vi "enqeue.vi"(9 "memory ref":refnum<k21>, 10 "data":u16, 11 "buffer state in":T1) -> (3 "buffer state out":T1)   [LabVIEW 2010, in "OnBoardBuffer.lvlib"]
uses:
  OnBoardBuffer.lvlib
  buffer_state_cluster.ctl
  <vilib>/rvi/DataTransferAndStorage/Container/XNode/niFpgaContainer.xnode
  <vilib>/rvi/DataTransferAndStorage/Container/Common/niFpgaContainerMetaDataKey.ctl
  <vilib>/rvi/DataTransferAndStorage/Container/Common/niFpgaContainerExecOnDevCompGetState.vi
  <vilib>/rvi/Memory/Memory_Emulation/nirvimemoryEmulationManagerCache_GetValue.vi
  <vilib>/rvi/DataTransferAndStorage/Container/Common/niFpgaContainerGetUniqueNameForEmu.vi
  <vilib>/rvi/Memory/Memory_Emulation/nirvimemoryEmulationManagerCache_InsertValue.vi
  <vilib>/Utility/error.llb/Clear Errors.vi
  <vilib>/rvi/Memory/Memory_Emulation/nirvimemoryEmulationManagerCache_SetValue.vi
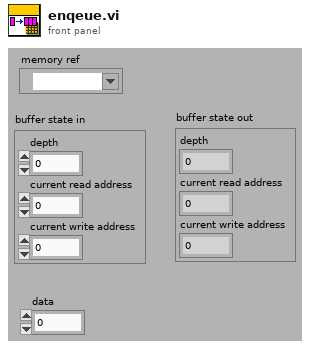
[diagram p1: front panel]
types:
  T1 = typedef "OnBoardBuffer.lvlib/buffer_state_cluster.ctl" = cluster{"depth":u32, "current read address":u32, "current write address":u32}
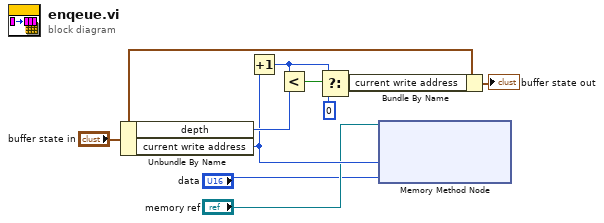
[diagram p0: block diagram]
diagram:
  n1 = Unbundle By Name("buffer state in") -> ("depth"=w10:u32, "current write address"=w3:u32)
  n2 = Increment(x=w3) -> (x+1=w7:u32)
  n3 = Less?(x=w7, y=w10) -> (x < y?=w9:bool)
  n4 = Select(t=w7, s=w9, f=u32 0) -> (s? t:f=w6:u32)
  n5 = Bundle By Name(cluster="buffer state in", "current write address"=w6) -> (→"buffer state out":T1)
  n6 = xnode ("Memory Method Node")("Address"=w3, "Data"="data", "Memory In"="memory ref") -> ()  [unwired: 1 out]
